vi "Read Show Panel User Event.vi"(8 "error in (no error)":errorcluster, 11 "Person in":refnum<class "Person.lvclass">) -> (0 "error out":errorcluster, 2 "Person Events":cluster{"Show Panel":refnum<user-event>}, 3 "Person out":refnum<class "Person.lvclass">)   [LabVIEW 2023, in "Person.lvlib" / "Person.lvclass"]
doc: "Read Person Events accessor VI"
uses:
  Person.lvclass
  Person.lvclass/Person.ctl
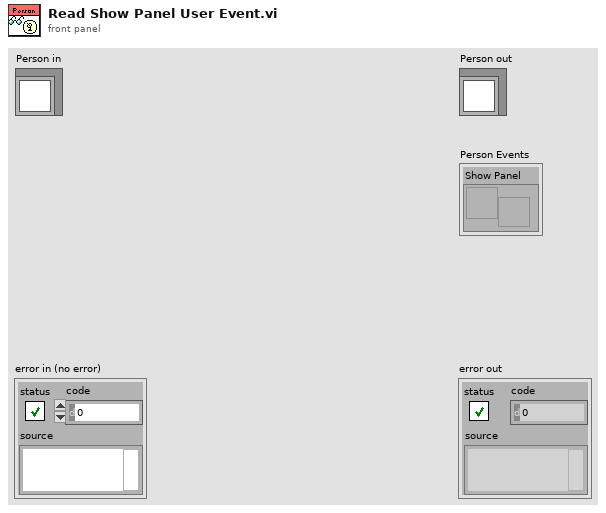
[diagram p1: front panel]
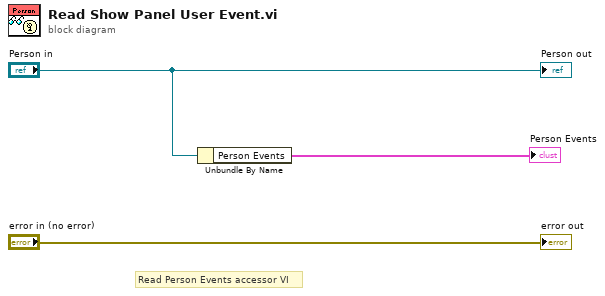
[diagram p0: block diagram]
diagram:
  # "Read Person Events accessor VI"
  n1 = Unbundle By Name("Person in") -> ("Person Events"=→"Person Events":cluster{"Show Panel":refnum<user-event>})
  "error out" <- "error in (no error)"
  "Person out" <- "Person in"
